vi "Address Based Construct.vi"(8 "error in":errorcluster, 9 "1553 address based handles":T1[](array[typedef]) {"acyclic frame trigger handles"."handle" format="%.0x"; "start stop handles"."stop handle" format="%.0x"; "start stop handles"."start handle" format="%.0x"}, 10 "biu configuration":T6, 11 "id":string) -> (0 "error out":errorcluster, 3 "Address Based Execution Unit Implementation out":refnum<class "Tx Acyclic Execution Unit.lvclass">)   [LabVIEW 2020, in "AIM MIL-STD-1553 Engine.lvlib" / "Implementation.lvlib" / "Tx Acyclic Execution Unit.lvclass"]
uses:
  Tx Acyclic Execution Unit.lvclass
  Execution Unit/Execution Unit.lvclass
  C:/dev/git/niveristand-aim-milStd1553-custom-device/Source/Custom Device Support/Engine/Implementation/Execution Unit/Execution Unit.lvclass
  C:/dev/git/niveristand-aim-milStd1553-custom-device/Source/Custom Device Support/Engine/Interfaces/Execution Unit/Execution Unit.lvclass
  C:/dev/git/niveristand-aim-milStd1553-custom-device/Source/Custom Device Support/Engine/Implementation/Address Based Execution Unit/Tx Acyclic Execution Unit.lvclass
  Shared/Address.ctl
  Shared/Terminal Endpoint.ctl
  Shared/Parameter Definition.ctl
  Shared/Message Type.ctl
  Shared/Message Definition.ctl
  Shared/BIU Configuration.ctl
  <vilib>/NI VeriStand/Custom Device API/Custom Device Item Ref.ctl
  <vilib>/NI VeriStand/Custom Device API/Custom Device API.lvlib
  Start Stop Channel Handles.ctl
  1553 Address Based Handles.ctl
  Acyclic Frame Trigger Handle.ctl
  Shared/Major Frame Definition.ctl
  Shared/Minor Frame Definition.ctl
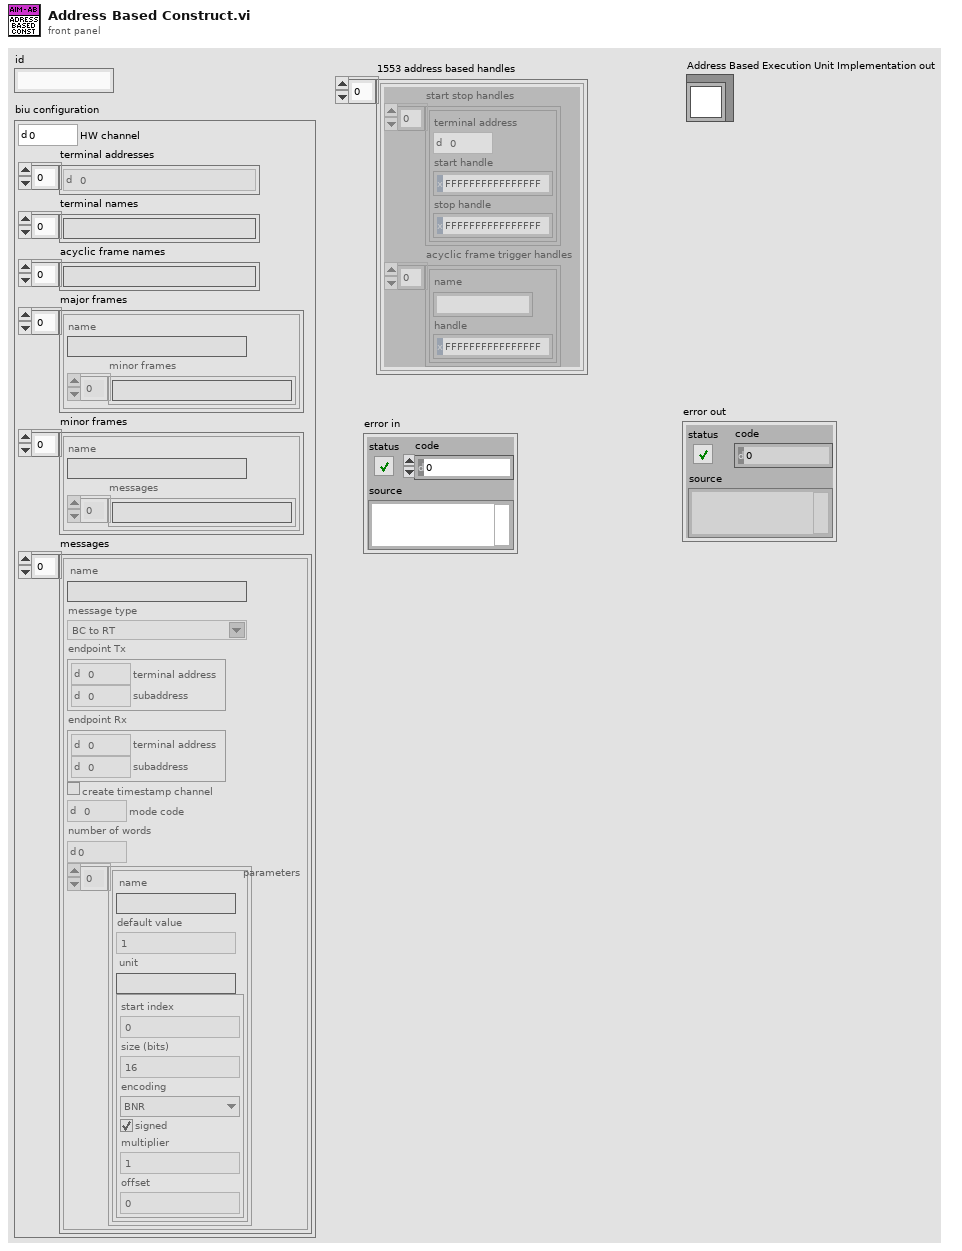
[diagram p1: front panel]
types:
  T1 = typedef "AIM MIL-STD-1553 Engine.lvlib/Implementation.lvlib/Tx Acyclic Execution Unit.lvclass/1553 Address Based Handles.ctl" = cluster{"start stop handles":T2[], "acyclic frame trigger handles":T5[]}
  T2 = typedef "AIM MIL-STD-1553 Engine.lvlib/Implementation.lvlib/Tx Acyclic Execution Unit.lvclass/Start Stop Channel Handles.ctl" = cluster{"terminal address":T3, "start handle":T4, "stop handle":T4}
  T3 = typedef "Address.ctl" = u16
  T4 = typedef "Custom Device API.lvlib/Custom Device Item Ref.ctl" = u64
  T5 = typedef "AIM MIL-STD-1553 Engine.lvlib/Implementation.lvlib/Tx Acyclic Execution Unit.lvclass/Acyclic Frame Trigger Handle.ctl" = cluster{"name":string, "handle":T4}
  T6 = typedef "BIU Configuration.ctl" = cluster{"HW channel":u16, "terminal addresses":T3[], "terminal names":string[], "acyclic frame names":string[], "major frames":T7[], "minor frames":T8[], "messages":T9[]}
  T7 = typedef "Major Frame Definition.ctl" = cluster{"name":string, "minor frames":string[]}
  T8 = typedef "Minor Frame Definition.ctl" = cluster{"name":string, "messages":string[]}
  T9 = typedef "Message Definition.ctl" = cluster{"name":string, "message type":T10, "endpoint Tx":T11, "endpoint Rx":T11, "create timestamp channel":bool, "mode code":u16, "number of words":u16, "parameters":cluster{"name":string, "default value":dbl, "unit":string, "parameter definition":T12}[]}
  T10 = typedef "Message Type.ctl" = string
  T11 = typedef "Terminal Endpoint.ctl" = cluster{"terminal address":T3, "subaddress":T3}
  T12 = typedef "Parameter Definition.ctl" = cluster{"start index":i32, "size (bits)":i32, "encoding":enum16{"BNR", "BCD", "Discrete"}, "signed":bool, "multiplier":dbl, "offset":dbl}
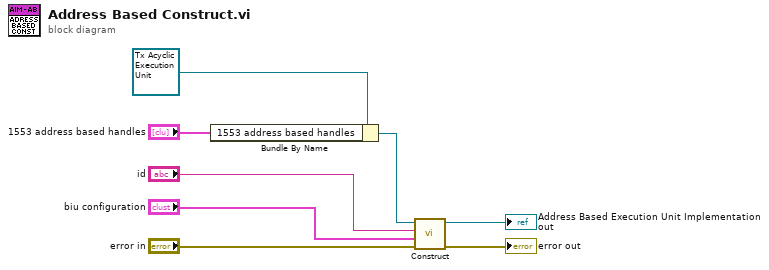
[diagram p0: block diagram]
diagram:
  n1 = Bundle By Name(cluster=refnum<class "Tx Acyclic Execution Unit.lvclass"> refnum ("Communication Bus Template Interfaces:Implementation.lvlib:Address Based Execution Unit.lvclass"), "1553 address based handles"="1553 address based handles") -> (w2:refnum<class "Tx Acyclic Execution Unit.lvclass">)
  n2 = call "Construct.vi"("error in"="error in", "biu configuration"="biu configuration", "id"="id", "execution unit"=w2) -> ("error out"=→"error out":errorcluster, "execution unit out"=→"Address Based Execution Unit Implementation out":refnum<class "Tx Acyclic Execution Unit.lvclass">)  [unwired: 6 in]
